vi "Wait Until Not Busy.vi"(6 "chip select (1st chip)":enum16{"1st chip", "2nd chip"}(ring), 8 "error in":errorcluster, 11 "HD44780 in":refnum<class "HD44780.lvclass">) -> (0 "error out":errorcluster, 3 "HD44780 out":refnum<class "HD44780.lvclass">)   [LabVIEW 2017, in "HD44780.lvclass"]
uses:
  HD44780.lvclass
  HD44780.lvclass/HD44780.ctl
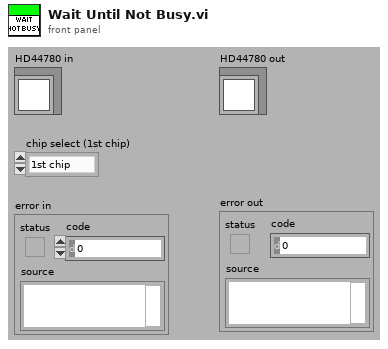
[diagram p1: front panel]
types:
  T1 = typedef "HD44780 Common.lvlib/cluster of class private data.ctl" = cluster{"FPGA VI Reference":refnum<k20>, "device index":i8, "screen size":T2, "font size":T3, "auto wrap":bool, "alignment":T4, "number of line":T5, "shift 0":i8, "entry mode 0":T6, "shift 1":i8, "entry mode 1":T6}
  T2 = typedef "HD44780 Common.lvlib/screen size.ctl" = enum8{"8x1", "8x2", "12x4", "16x1", "16x2", "16x4", "20x1", "20x2", "20x4", "24x1", "24x2", "40x2", "40x4"}
  T3 = typedef "HD44780 Common.lvlib/font size.ctl" = enum8{"5x8", "5x10"}
  T4 = typedef "HD44780 Common.lvlib/alignment.ctl" = enum16{"None", "Left", "Center", "Right"}
  T5 = typedef "HD44780 Common.lvlib/line number.ctl" = enum8{"1 line", "2 lines"}
  T6 = typedef "HD44780 Common.lvlib/entry mode.ctl" = enum8{"increment & no shift", "increment & shift", "decrement & no shift", "decrement & shift"}
  T7 = cluster{"FPGA VI Reference":refnum<k20>, "device index":i8, "screen size":enum8{"8x1", "8x2", "12x4", "16x1", "16x2", "16x4", "20x1", "20x2", "20x4", "24x1", "24x2", "40x2", "40x4"}, "font size":enum8{"5x8", "5x10"}, "auto wrap":bool, "alignment":enum16{"None", "Left", "Center", "Right"}, "number of line":enum8{"1 line", "2 lines"}, "shift 0":i8, "entry mode 0":enum8{"increment & no shift", "increment & shift", "decrement & no shift", "decrement & shift"}, "shift 1":i8, "entry mode 1":enum8{"increment & no shift", "increment & shift", "decrement & no shift", "decrement & shift"}}
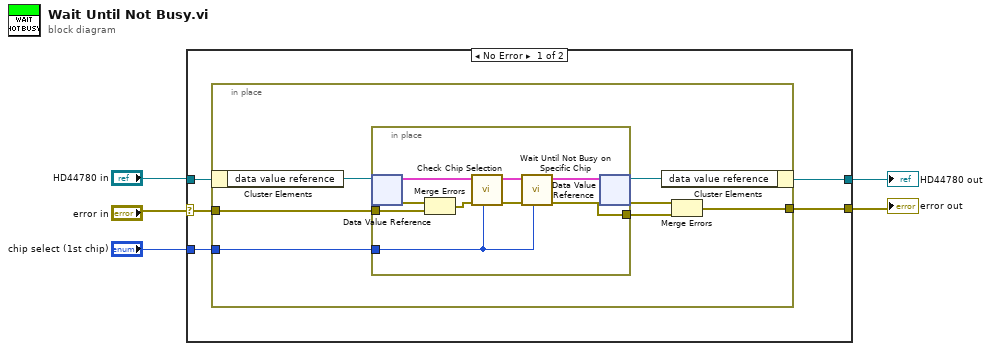
[diagram p0: block diagram]
diagram:
  n1 = case shown="No Error" "error in" {
    selector: "error in" -> [w7 w28]
    tunnel: "HD44780 in" -> [w10 w27]
    tunnel: [w9 w27] -> w4
    tunnel: [w8 w28] -> w2
    tunnel: "chip select (1st chip)" -> [w6 _]
    frame No Error {
      n2 = in-place {
        in-place-border: [w13] -> w8
        in-place-border: w7 -> [w12]
        in-place-border: w6 -> [w11]
        n3 = in-place-cluster #1(w10) -> ("data value reference"=w17:refnum<data-value>)
        n4 = in-place {
          in-place-border: [w25] -> w14
          in-place-border: w12 -> [w23]
          in-place-border: w11 -> [w18]
          n5 = in-place-dvr #2(w17) -> (w21:T1, w24:errorcluster)
          n6 = Merge Errors(w24, w23) -> (w22:errorcluster)
          n7 = call "Check Chip Selection.vi"("chip select"=w18, "error in (no error)"=w22, "cluster of private data in"=w21) -> ("error out"=w20:errorcluster, "cluster of private data out"=w19:T7)  [unwired: 7 in]
          n8 = call "Wait Until Not Busy on Specific Chip.vi"("chip select  (1st chip)"=w18, "error in (no error)"=w20, "cluster of private data in"=w19) -> ("error out"=w25:errorcluster, "cluster of private data out"=w26:T7)  [unwired: 7 in]
          n9 = in-place-dvr #2(w26) -> (w15:refnum<data-value>, w16:errorcluster)
        }
        n10 = in-place-cluster #1("data value reference"=w15) -> (w9:refnum<class "HD44780.lvclass">)
        n11 = Merge Errors(w16, w14) -> (w13:errorcluster)
      }
    }
    frame Error {
    }
  }
  "HD44780 out" <- w4
  "error out" <- w2
